vi "Position_raw.vi"(11 "Shift":dbl) -> (1 "Z":dbl, 2 "Y":dbl, 3 "X":dbl)   [LabVIEW 2019]
uses:
  <userlib>/HapticSTM/HapticSTM.lvlib
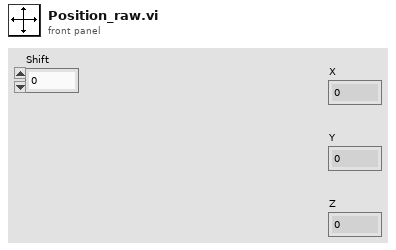
[diagram p1: front panel]
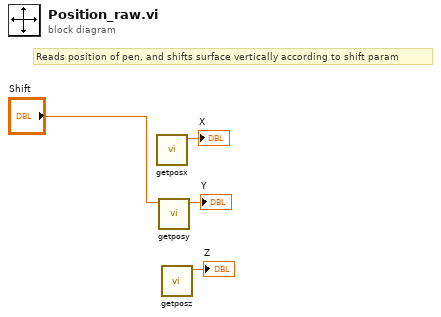
[diagram p0: block diagram]
diagram:
  # "Reads position of pen, and shifts surface vertically according to shift param"
  n1 = call <userlib>:"getposx.vi"() -> ("function return"=→"X":dbl)  [unwired: 11 in]
  n2 = call <userlib>:"getposy.vi"("shift"="Shift") -> ("function return"=→"Y":dbl)  [unwired: 10 in]
  n3 = call <userlib>:"getposz.vi"() -> ("function return"=→"Z":dbl)  [unwired: 11 in]
